vi "Close.vi"(8 "error in":errorcluster, 11 "Chiller in":refnum<class "Chiller.lvclass">) -> (0 "error out":errorcluster, 3 "Chiller out":refnum<class "Chiller.lvclass">)   [LabVIEW 2023, in "Chiller.lvclass"]
uses:
  Chiller.lvclass
  Chiller.lvclass/Chiller.ctl
  Low Level Capabilities/OnOff/OnOff.lvclass
  Low Level Capabilities/Error Channels/Error Channels.lvclass
  Low Level Capabilities/Temperature/Temperature Gradient/Temperature Gradient.lvclass
  Low Level Capabilities/Temperature/Temperature Limit/Temperature Limit.lvclass
  Low Level Capabilities/Temperature/Temperature Setpoint/Temperature Setpoint.lvclass
  Low Level Capabilities/Pressure/Pressure Gradient/Pressure Gradient.lvclass
  Low Level Capabilities/Pressure/Pressure Limit/Pressure Limit.lvclass
  Low Level Capabilities/Pressure/Pressure Setpoint/Pressure Setpoint.lvclass
  Low Level Capabilities/Flow/Flow Actual Value/Flow Actual Value.lvclass
  Low Level Capabilities/Flow/Flow Gradient/Flow Gradient.lvclass
  Low Level Capabilities/Flow/Flow Limit/Flow Limit.lvclass
  Low Level Capabilities/Flow/Flow Setpoint/Flow Setpoint.lvclass
  Low Level Capabilities/Control Mode/Control Mode.lvclass
  Low Level Capabilities/Pressure/Pressure Actual Value/Pressure Actual Value.lvclass
  Low Level Capabilities/Temperature/Temperature Actual Value/Temperature Actual Value.lvclass
  Low Level Capabilities/Error/Error.lvclass
  Low Level Capabilities/Output Enable/Output Enable.lvclass
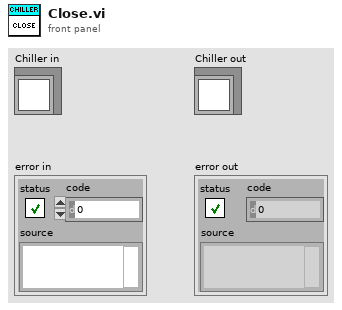
[diagram p1: front panel]
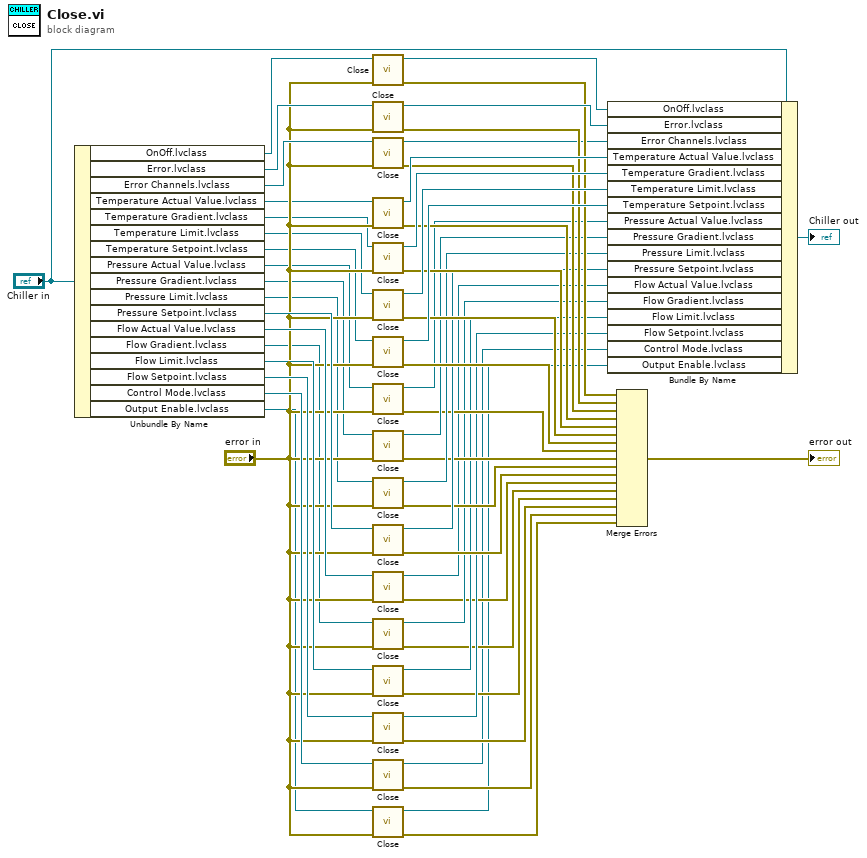
[diagram p0: block diagram]
diagram:
  n1 = Unbundle By Name("Chiller in") -> ("OnOff.lvclass"=w53:refnum<class "OnOff.lvclass">, "Error.lvclass"=w51:refnum<class "Error.lvclass">, "Error Channels.lvclass"=w39:refnum<class "Error Channels.lvclass">, "Temperature Actual Value.lvclass"=w8:refnum<class "Temperature Actual Value.lvclass">, "Temperature Gradient.lvclass"=w7:refnum<class "Temperature Gradient.lvclass">, "Temperature Limit.lvclass"=w6:refnum<class "Temperature Limit.lvclass">, "Temperature Setpoint.lvclass"=w5:refnum<class "Temperature Setpoint.lvclass">, "Pressure Actual Value.lvclass"=w4:refnum<class "Pressure Actual Value.lvclass">, "Pressure Gradient.lvclass"=w3:refnum<class "Pressure Gradient.lvclass">, "Pressure Limit.lvclass"=w2:refnum<class "Pressure Limit.lvclass">, "Pressure Setpoint.lvclass"=w32:refnum<class "Pressure Setpoint.lvclass">, "Flow Actual Value.lvclass"=w27:refnum<class "Flow Actual Value.lvclass">, "Flow Gradient.lvclass"=w10:refnum<class "Flow Gradient.lvclass">, "Flow Limit.lvclass"=w26:refnum<class "Flow Limit.lvclass">, "Flow Setpoint.lvclass"=w25:refnum<class "Flow Setpoint.lvclass">, "Control Mode.lvclass"=w14:refnum<class "Control Mode.lvclass">, "Output Enable.lvclass"=w11:refnum<class "Output Enable.lvclass">)
  n2 = call-dynamic "Close.vi"("error in"="error in", "OnOff in"=w53) -> ("error out"=w45:errorcluster, "OnOff out"=w52:refnum<class "OnOff.lvclass">)  [unwired: 8 in]
  n3 = call-dynamic "Close.vi"("error in"="error in", "Error in"=w51) -> ("error out"=w44:errorcluster, "Error out"=w50:refnum<class "Error.lvclass">)  [unwired: 8 in]
  n4 = call-dynamic "Close.vi"("error in"="error in", "Error Channels in"=w39) -> ("error out"=w37:errorcluster, "Error Channels out"=w38:refnum<class "Error Channels.lvclass">)  [unwired: 8 in]
  n5 = call-dynamic "Close.vi"("error in"="error in", "Temperature Actual Value in"=w8) -> ("error out"=w43:errorcluster, "Temperature Actual Value out"=w49:refnum<class "Temperature Actual Value.lvclass">)  [unwired: 8 in]
  n6 = call-dynamic "Close.vi"("error in"="error in", "Temperature Gradient in"=w7) -> ("error out"=w42:errorcluster, "Temperature Gradient out"=w47:refnum<class "Temperature Gradient.lvclass">)  [unwired: 8 in]
  n7 = call-dynamic "Close.vi"("error in"="error in", "Temperature Limit in"=w6) -> ("error out"=w41:errorcluster, "Temperature Limit out"=w46:refnum<class "Temperature Limit.lvclass">)  [unwired: 8 in]
  n8 = call-dynamic "Close.vi"("error in"="error in", "Temperature Setpoint in"=w5) -> ("error out"=w40:errorcluster, "Temperature Setpoint out"=w48:refnum<class "Temperature Setpoint.lvclass">)  [unwired: 8 in]
  n9 = call-dynamic "Close.vi"("error in"="error in", "Pressure Actual Value in"=w4) -> ("error out"=w31:errorcluster, "Pressure Actual Value out"=w36:refnum<class "Pressure Actual Value.lvclass">)  [unwired: 8 in]
  n10 = call-dynamic "Close.vi"("error in"="error in", "Pressure Gradient in"=w3) -> ("error out"=w30:errorcluster, "Pressure Gradient out"=w35:refnum<class "Pressure Gradient.lvclass">)  [unwired: 8 in]
  n11 = call-dynamic "Close.vi"("error in"="error in", "Pressure Limit in"=w2) -> ("error out"=w29:errorcluster, "Pressure Limit out"=w34:refnum<class "Pressure Limit.lvclass">)  [unwired: 8 in]
  n12 = call-dynamic "Close.vi"("error in"="error in", "Pressure Setpoint in"=w32) -> ("error out"=w28:errorcluster, "Pressure Setpoint out"=w33:refnum<class "Pressure Setpoint.lvclass">)  [unwired: 8 in]
  n13 = call-dynamic "Close.vi"("error in"="error in", "Flow Actual Value in"=w27) -> ("error out"=w20:errorcluster, "Flow Actual Value out"=w24:refnum<class "Flow Actual Value.lvclass">)  [unwired: 8 in]
  n14 = call-dynamic "Close.vi"("error in"="error in", "Flow Gradient in"=w10) -> ("error out"=w19:errorcluster, "Flow Gradient out"=w23:refnum<class "Flow Gradient.lvclass">)  [unwired: 8 in]
  n15 = call-dynamic "Close.vi"("error in"="error in", "Flow Limit in"=w26) -> ("error out"=w18:errorcluster, "Flow Limit out"=w22:refnum<class "Flow Limit.lvclass">)  [unwired: 8 in]
  n16 = call-dynamic "Close.vi"("error in"="error in", "Flow Setpoint in"=w25) -> ("error out"=w17:errorcluster, "Flow Setpoint out"=w21:refnum<class "Flow Setpoint.lvclass">)  [unwired: 8 in]
  n17 = call-dynamic "Close.vi"("error in"="error in", "Control Mode in"=w14) -> ("error out"=w16:errorcluster, "Control Mode out"=w15:refnum<class "Control Mode.lvclass">)  [unwired: 8 in]
  n18 = call-dynamic "Close.vi"("error in"="error in", "Output Enable in"=w11) -> ("error out"=w12:errorcluster, "Output Enable out"=w1:refnum<class "Output Enable.lvclass">)  [unwired: 8 in]
  n19 = Bundle By Name(cluster="Chiller in", "OnOff.lvclass"=w52, "Error.lvclass"=w50, "Error Channels.lvclass"=w38, "Temperature Actual Value.lvclass"=w49, "Temperature Gradient.lvclass"=w47, "Temperature Limit.lvclass"=w46, "Temperature Setpoint.lvclass"=w48, "Pressure Actual Value.lvclass"=w36, "Pressure Gradient.lvclass"=w35, "Pressure Limit.lvclass"=w34, "Pressure Setpoint.lvclass"=w33, "Flow Actual Value.lvclass"=w24, "Flow Gradient.lvclass"=w23, "Flow Limit.lvclass"=w22, "Flow Setpoint.lvclass"=w21, "Control Mode.lvclass"=w15, "Output Enable.lvclass"=w1) -> (→"Chiller out":refnum<class "Chiller.lvclass">)
  n20 = Merge Errors(w45, w44, w37, w43, w42, w41, w40, w31, w30, w29, w28, w20, w19, w18, w17, w16, w12) -> (→"error out":errorcluster)
